vi "AI Table Read.vi"(8 "error in (no error)":errorcluster caption="错误输入（无错误）", 10 "Task":string="AO", 11 "Read Path":path) -> (0 "error out":errorcluster caption="错误输出", 1 "ItemNames":string[][](array[string]), 3 "TaskParam":T1[](array[typedef]), 4 "ColHdrString":string[](array[string]))   [LabVIEW 2013]
uses:
  AI Param.ctl
  MeasurementType.ctl
  AI Terminal Configuration.ctl
  <vilib>/Utility/sysdir.llb/System Directory Type.ctl
  <vilib>/Utility/VariantDataType/VariantType.lvlib
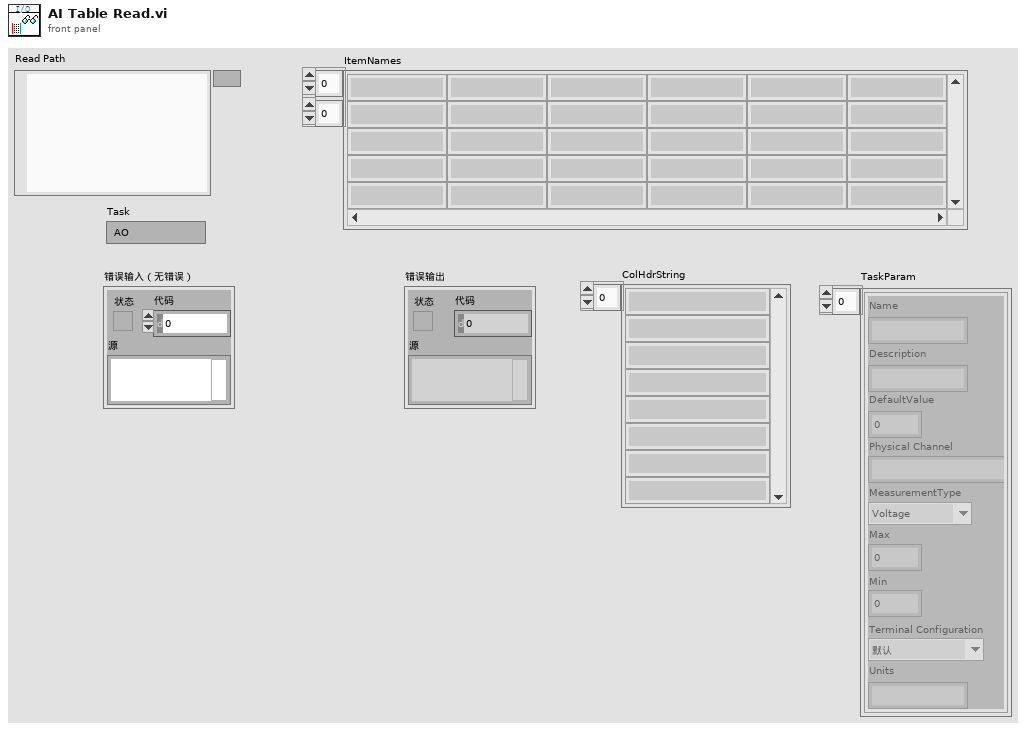
[diagram p1: front panel]
types:
  T1 = typedef "AI Param.ctl" = cluster{"Name":string, "Description":string, "DefaultValue":dbl, "Physical Channel":string, "MeasurementType":T2, "Max":dbl, "Min":dbl, "Terminal Configuration":T3, "Units":string}
  T2 = typedef "MeasurementType.ctl" = enum16{"Voltage", "Current", "More:Voltage:Custom with Excitation", "More:Current:Custom with Excitation", "Frequency", "Period", "Resistance", "Temperature:Thermocouple", "Temperature:Thermistor", "Temperature:RTD", "Temperature:Built-in Sensor", "Strain Gage"}
  T3 = typedef "AI Terminal Configuration.ctl" = enum16{"默认", "RSE", "NRSE", "差分", "伪差分"}
  T4 = typedef "System Directory Type.ctl" = i32
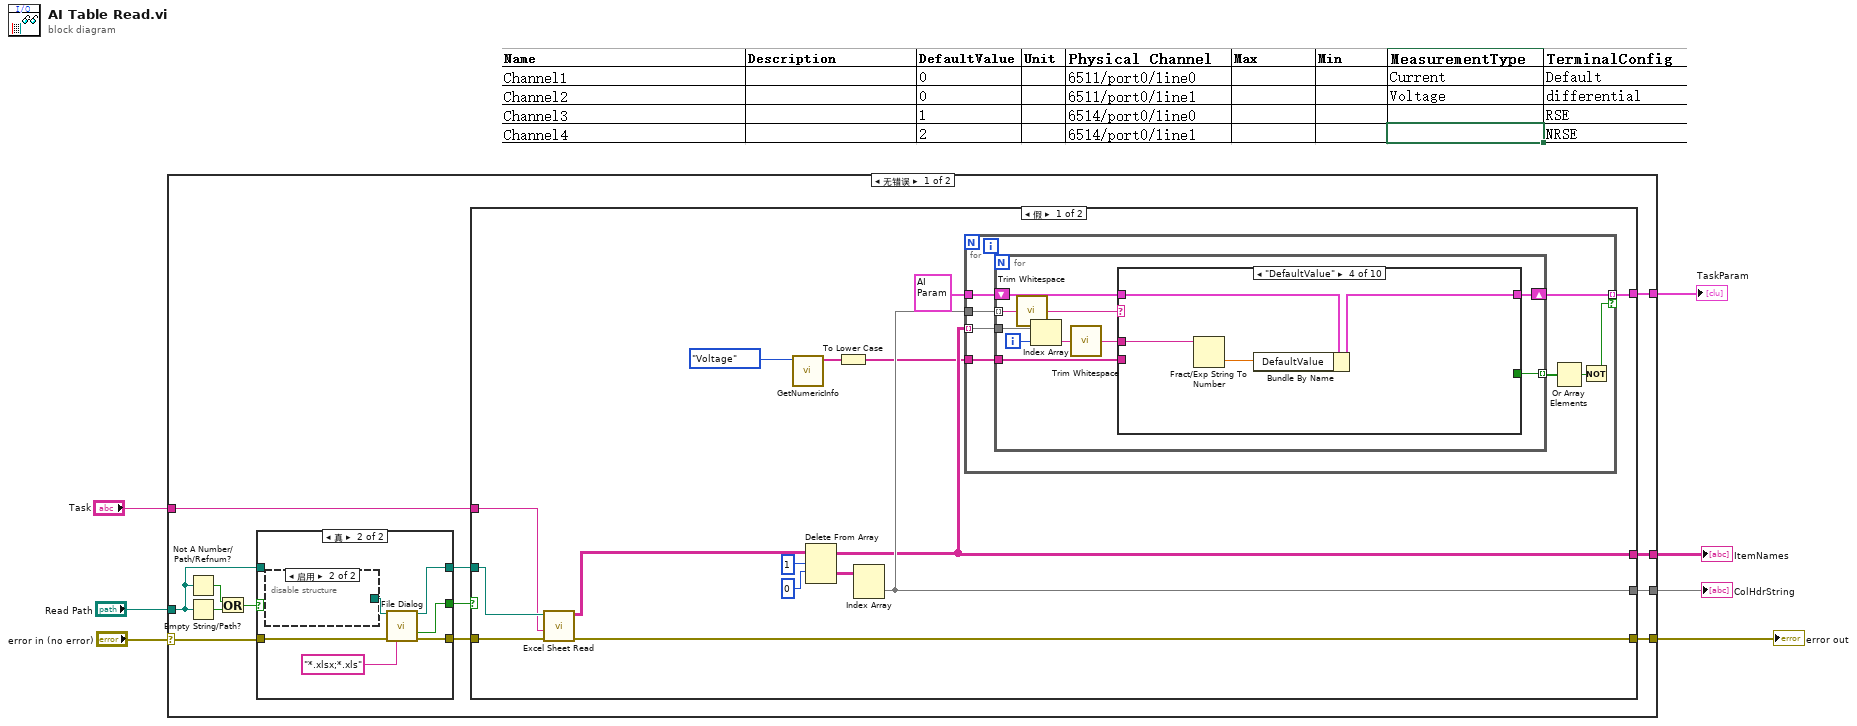
[diagram p0: block diagram]
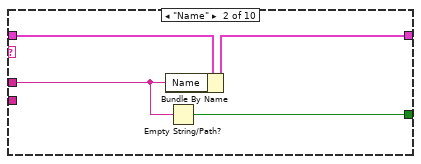
[diagram p3: hidden frame]
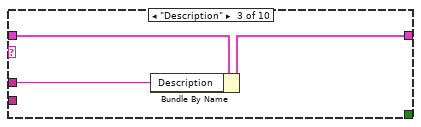
[diagram p4: hidden frame]
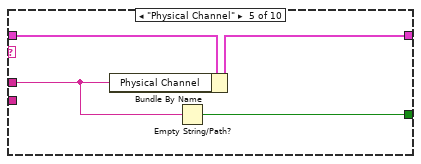
[diagram p5: hidden frame]
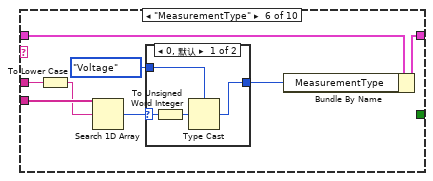
[diagram p6: hidden frame]
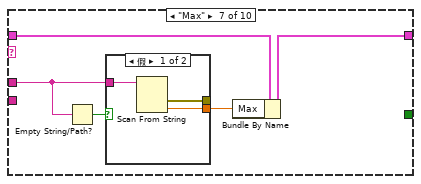
[diagram p8: hidden frame]
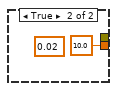
[diagram p9: hidden frame]
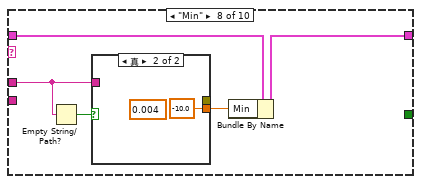
[diagram p10: hidden frame]
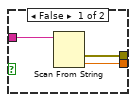
[diagram p11: hidden frame]
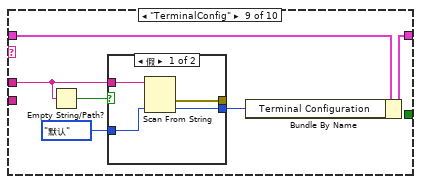
[diagram p12: hidden frame]
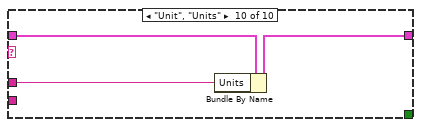
[diagram p14: hidden frame]
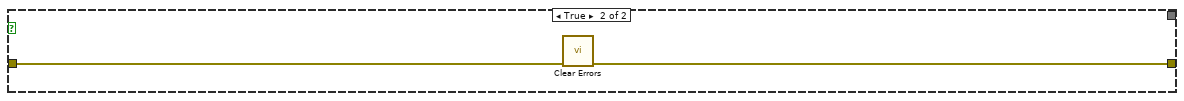
[diagram p15: hidden frame]
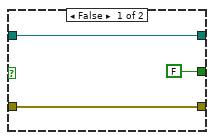
[diagram p16: hidden frame]
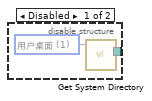
[diagram p17: hidden frame]
diagram:
  n1 = case shown="无错误" "error in (no error)" {
    selector: "error in (no error)" -> [w14 w128]
    tunnel: "Read Path" -> [w12 _]
    tunnel: [w20 w128] -> w6
    tunnel: [w19 _] -> w5
    tunnel: [w18 _] -> w4
    tunnel: "Task" -> [w9 _]
    tunnel: [w8 _] -> w1
    frame No Error {
      n2 = Not A Number/Path/Refnum?(number/path/refnum=w12) -> (NaN/Path/Refnum?=w15:bool)
      n3 = Empty String/Path?(string/path=w12) -> (empty?=w16:bool)
      n4 = Or(x=w15, y=w16) -> (x .or. y?=w17:bool)
      n5 = case shown="真" w17 {
        tunnel: w14 -> [w119 w125]
        tunnel: [w119 w124] -> w13
        tunnel: [w118 w123] -> w11
        tunnel: w12 -> [w118 _]
        tunnel: [FALSE ("cancelled") w121] -> w10
        frame False {
        }
        frame True {
          n6 = disable-structure shown="启用" {
            disable-tunnel: [w126 _] -> w120
            frame Disabled {
              w127 = T4 1 items=["用户目录"=0, "用户桌面"=1, "用户文档"=2, "用户应用程序数据"=3, "用户设置"=4, "用户临时目录"=5, "公共文档"=6, "公共应用程序数据"=7, "公共设置"=8, "公共缓存"=13, "系统核心库"=9, "系统安装库"=10, "应用程序文件"=11, "启动盘根目录"=12] ("system directory type")
              n7 = call <vilib>:"Get System Directory.vi"("system directory type"=w127) -> ("system directory"=w126:path)  [unwired: 10 in]
            }
            frame Enabled {
            }
          }
          n8 = call "File Dialog"("start path"=w120, "error in"=w125, "pattern (all files)"="*.xlsx;*.xls") -> ("selected path"=w123:path, "cancelled"=w121:bool, "error out"=w124:errorcluster)  [unwired: 4 in, 6 out]
        }
      }
      n9 = case shown="假" w10 {
        tunnel: [w25 w115] -> w20
        tunnel: [w30 _] -> w19
        tunnel: [w24 _] -> w18
        tunnel: w13 -> [w28 w116]
        tunnel: w11 -> [w29 _]
        tunnel: w9 -> [w27 _]
        tunnel: [w31 _] -> w8
        frame False {
          n10 = call "Excel Sheet Read.vi"("error in (no error)"=w28, "Name(\"\")"=w27, "Excel Path"=w29) -> ("error out"=w25:errorcluster, "Data"=w26:string[][])  [unwired: 7 in]
          n11 = call <vilib>:"GetNumericInfo.vi"("Variant"=MeasurementType."Voltage" ("MeasurementType")) -> ("EnumNames"=w23:string[])  [unwired: 7 in, 3 out]
          n12 = Delete From Array(array=w26, length=1 ("长度"), index (row)=0 ("索引 (行)")) -> (deleted portion=w33:string[][], array with subset deleted=w24:string[][])  [unwired: 1 in]
          n13 = To Lower Case(string=w23) -> (all lower case string=w22:string[])
          n14 = Index Array(array=w33) -> (element=w30:string[])  [unwired: 2 in]
          n15 = for {
            tunnel: w24 -> [w40] mode=indexing
            tunnel: T1 {"Name"="", "Description"="", "DefaultValue"=0.0, "Physical Channel"="", "MeasurementType"=enum."Voltage", "Max"=0.0, "Min"=0.0, "Terminal Configuration"=enum."默认", "Units"=""} ("Task") -> [w42]
            tunnel: w30 -> [w43]
            tunnel: [w41] -> w31 mode=indexing if=w36
            tunnel: w22 -> [w39]
            n16 = for {
              tunnel: w43 -> [w53] mode=indexing
              shift-right: [w51] -> w41
              shift-left: w42 -> [w52]
              tunnel: w40 -> [w49]
              tunnel: w39 -> [w47]
              tunnel: [w44] -> w38 mode=indexing
              i -> [w50]
              n17 = call <vilib>:"Trim Whitespace.vi"("string"=w53) -> ("trimmed string"=w46:string)  [unwired: 1 in]
              n18 = Index Array(array=w49, index=w50) -> (element=w48:string)
              n19 = call <vilib>:"Trim Whitespace.vi"("string"=w48) -> ("trimmed string"=w45:string)  [unwired: 1 in]
              n20 = case shown="\"DefaultValue\"" w46 {
                tunnel: w52 -> [w54 w58 w61 w65 w69 w77 w87 w96 w106 w114]
                tunnel: [w54 w57 w60 w64 w68 w76 w86 w95 w105 w113] -> w51
                tunnel: w45 -> [_ w56 w59 w62 w67 w74 w83 w92 w103 w112]
                tunnel: w47 -> [_ _ _ _ _ w75 _ _ _ _]
                tunnel: [_ w55 _ _ w66 _ _ _ _ _] -> w44
                frame Default {
                }
                frame "Name" {
                  n21 = Bundle By Name(cluster=w58, "Name"=w56) -> (w57:T1)
                  n22 = Empty String/Path?(string/path=w56) -> (empty?=w55:bool)
                }
                frame "Description" {
                  n23 = Bundle By Name(cluster=w61, "Description"=w59) -> (w60:T1)
                }
                frame "DefaultValue" {
                  n24 = Fract/Exp String To Number(string=w62) -> (number=w63:dbl)  [unwired: 3 in, 1 out]
                  n25 = Bundle By Name(cluster=w65, "DefaultValue"=w63) -> (w64:T1)
                }
                frame "Physical Channel" {
                  n26 = Bundle By Name(cluster=w69, "Physical Channel"=w67) -> (w68:T1)
                  n27 = Empty String/Path?(string/path=w67) -> (empty?=w66:bool)
                }
                frame "MeasurementType" {
                  n28 = To Lower Case(string=w74) -> (all lower case string=w73:string)
                  n29 = Search 1D Array(1D array=w75, element=w73) -> (index of element=w72:i32)  [unwired: 1 in]
                  n30 = case shown="0, 默认" w72 {
                    selector: w72 -> [w81 _]
                    tunnel: MeasurementType."Voltage" ("MeasurementType") -> [w80 w82]
                    tunnel: [w79 w82] -> w71
                    frame 0, Default {
                      n31 = To Unsigned Word Integer(number=w81) -> (unsigned 16bit integer=w78:u16)
                      n32 = Type Cast(type=w80, x=w78) -> (*(type *) &x=w79:T2)
                    }
                    frame -1 {
                    }
                  }
                  n33 = Bundle By Name(cluster=w77, "MeasurementType"=w71) -> (w76:T1)
                }
                frame "Max" {
                  n34 = Empty String/Path?(string/path=w83) -> (empty?=w85:bool)
                  n35 = case shown="假" w85 {
                    tunnel: [w89 10.0 ("Max")] -> w84
                    tunnel: w83 -> [w90 _]
                    tunnel: [w88 _] -> _
                    frame False {
                      n36 = Scan From String(input string=w90) -> (error out=w88:errorcluster, output 1=w89:dbl)  [unwired: 4 in, 2 out]
                    }
                    frame True {
                      (unwired) 0.02 ("Max")
                    }
                  }
                  n37 = Bundle By Name(cluster=w87, "Max"=w84) -> (w86:T1)
                }
                frame "Min" {
                  n38 = Empty String/Path?(string/path=w92) -> (empty?=w94:bool)
                  n39 = case shown="真" w94 {
                    tunnel: [w98 -10.0 ("Max")] -> w93
                    tunnel: w92 -> [w99 _]
                    tunnel: [w97 _] -> _
                    frame False {
                      n40 = Scan From String(input string=w99) -> (error out=w97:errorcluster, output 1=w98:dbl)  [unwired: 4 in, 2 out]
                    }
                    frame True {
                      (unwired) 0.004 ("Max")
                    }
                  }
                  n41 = Bundle By Name(cluster=w96, "Min"=w93) -> (w95:T1)
                }
                frame "TerminalConfig" {
                  n42 = Empty String/Path?(string/path=w103) -> (empty?=w104:bool)
                  n43 = case shown="假" w104 {
                    tunnel: [w107 w111] -> w102
                    tunnel: w103 -> [w110 _]
                    tunnel: [w109 _] -> _
                    tunnel: AI_Terminal_Configuration."默认" ("Terminal Configuration") -> [w108 w111]
                    frame False {
                      n44 = Scan From String(input string=w110, default 1=w108) -> (error out=w109:errorcluster, output 1=w107:T3)  [unwired: 3 in, 2 out]
                    }
                    frame True {
                    }
                  }
                  n45 = Bundle By Name(cluster=w106, "Terminal Configuration"=w102) -> (w105:T1)
                }
                frame "Unit", "Units" {
                  n46 = Bundle By Name(cluster=w114, "Units"=w112) -> (w113:T1)
                }
              }
            }
            n47 = Or Array Elements(Boolean array=w38) -> (logical OR=w37:bool)
            n48 = Not(x=w37) -> (.not. x?=w36:bool)
          }
        }
        frame True {
          n49 = call <vilib>:"Clear Errors.vi"("error in (no error)"=w116) -> ("error out"=w115:errorcluster)  [unwired: 6 in]
        }
      }
    }
    frame Error {
    }
  }
  "ItemNames" <- w4
  "error out" <- w6
  "ColHdrString" <- w5
  "TaskParam" <- w1
